vi "draw ROI on intensity plot.vi"(6 "Intensity array in":u64[][](array[numeric]), 7 "mouse positon":cluster{"X":dbl, "Y":dbl}, 8 "error in (no error)":errorcluster, 9 "draw gate? in":bool, 10 "y array in":dbl[](array[numeric]), 11 "x array in":dbl[](array[numeric])) -> (0 "error out":errorcluster, 1 "draw gate out":bool, 2 "y array out":dbl[](array[numeric]), 3 "x array out":dbl[](array[numeric]), 4 "intensity array out":u64[][](array[numeric]))   [LabVIEW 2016]
doc: "If ROI is being drawn, this vi takes the mouses location and generates a viewable\ngate."
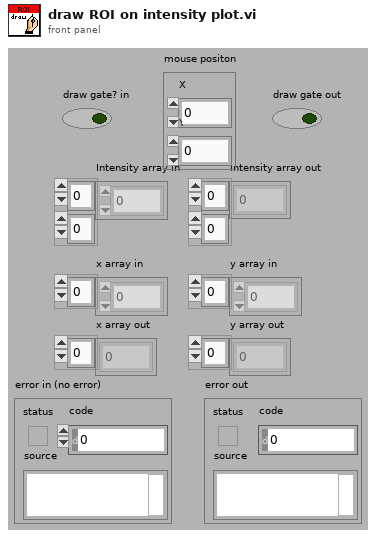
[diagram p1: front panel]
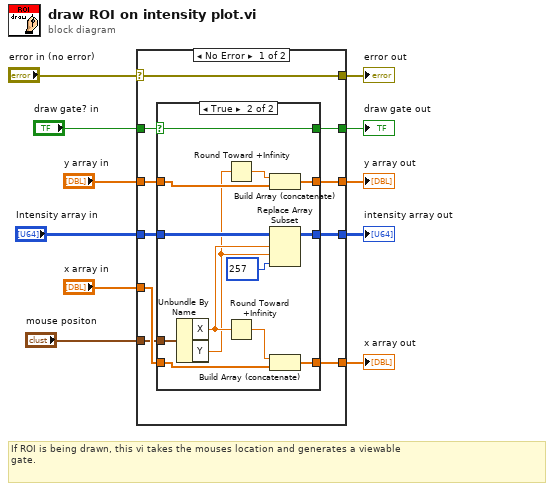
[diagram p0: block diagram]
diagram:
  # "If ROI is being drawn, this vi takes the mouses location and generates a viewable\ngate."
  n1 = case shown="No Error" "error in (no error)" {
    selector: "error in (no error)" -> [w12 w39]
    tunnel: [w21 w42] -> w11
    tunnel: "Intensity array in" -> [w20 w42]
    tunnel: [w19 w43] -> w9
    tunnel: "draw gate? in" -> [w18 w43]
    tunnel: "y array in" -> [w17 w40]
    tunnel: "x array in" -> [w16 w41]
    tunnel: [w15 w40] -> w5
    tunnel: [w14 w41] -> w4
    tunnel: "mouse positon" -> [w13 _]
    tunnel: [w12 w39] -> w1
    frame No Error {
      n2 = case shown="True" w18 {
        selector: w18 -> [w22 w30]
        tunnel: w20 -> [w25 w37]
        tunnel: w13 -> [_ w38]
        tunnel: [w25 w35] -> w21
        tunnel: [w24 w34] -> w14
        tunnel: [w23 w33] -> w15
        tunnel: w16 -> [w24 w32]
        tunnel: w17 -> [w23 w31]
        tunnel: [w22 w30] -> w19
        frame False {
        }
        frame True {
          n3 = Unbundle By Name(w38) -> ("X"=w29:dbl, "Y"=w27:dbl)
          n4 = Round Toward +Infinity(x=w27) -> (ceil(x): smallest int >= x=w26:dbl)
          n5 = Round Toward +Infinity(x=w29) -> (ceil(x): smallest int >= x=w28:dbl)
          n6 = Build Array (concatenate)(w26, w31) -> (w33:dbl[])
          n7 = Replace Array Subset(array=w37, new element=257 ("new element/subarray"), index (row)=w29, index (col)=w27) -> (w35:u64[][])
          n8 = Build Array (concatenate)(w28, w32) -> (w34:dbl[])
        }
      }
    }
    frame Error {
    }
  }
  "intensity array out" <- w11
  "draw gate out" <- w9
  "y array out" <- w5
  "x array out" <- w4
  "error out" <- w1
